vi "SENS_IF_FILT_STAG_TYPE.vi"(0 "VISA IN":refnum<visa-resource-name>, 1 "Filter Type":string, 5 "error in":errorcluster, 7 "Channel":i32) -> (14 "VISA Out":refnum<visa-resource-name>, 19 "error out":errorcluster)   [LabVIEW 2018, in "PNA-X.lvlib"]
doc: "SENSe<cnum>:IF:FILTer:STAGe3:TYPE <value> \n(Read-Write) Sets and returns the Stage 3 filter type. This command is only used when \nSENSe:IF:FILTer:AUTO is set to False (Manual). \nCritical Note \nParameters \n<cnum> Existing channel number. If unspecified, <cnum> is set to 1. \n<value> (String) Filter type. Chose from: \n\"RECT\" Rectangular Window Filter \n\"TUKEY\" Tukey Filter \n\"PWIN\" Pulse Window Filter \nExamples SENS:IF:FILT:STAGe3:TYPE RECT \nsense2:if:filter:stage3:type pwin \nQuery Syntax SENSe<cnum>:IF:FILTer:STAGE3:TYPE? \nReturn Type String \nDefault \"TUKEY\""
uses:
  PNA-X.lvlib
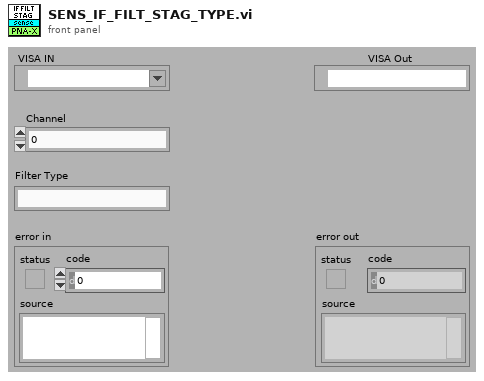
[diagram p1: front panel]
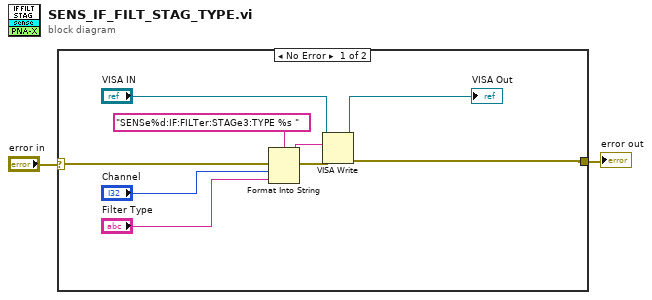
[diagram p0: block diagram]
diagram:
  n1 = case shown="No Error" "error in" {
    selector: "error in" -> [w11 w12]
    tunnel: [w6 w12] -> w1
    frame No Error {
      n2 = Format Into String(format string="SENSe%d:IF:FILTer:STAGe3:TYPE %s " ("Cmdline"), error in=w11, "Channel", "Filter Type") -> (resulting string=w9:string, error out=w10:errorcluster)  [unwired: 1 in]
      n3 = VISA Write(VISA resource name="VISA IN", write buffer=w9, error in (no error)=w10) -> (VISA resource name out=→"VISA Out":refnum<visa-resource-name>, error out=w6:errorcluster)  [unwired: 1 out]
    }
    frame Error {
    }
  }
  "error out" <- w1
